vi "mxwScript_API_XMLTemplateName_AddCreateSpace.vi"(8 "error in (no error)":errorcluster, 10 "createSpace?":bool=TRUE, 11 "absolutePath":string) -> (0 "error out":errorcluster, 3 "encoded absolutePath":string)   [LabVIEW 2017]
doc: "Add diagram to drop this template into to the template name."
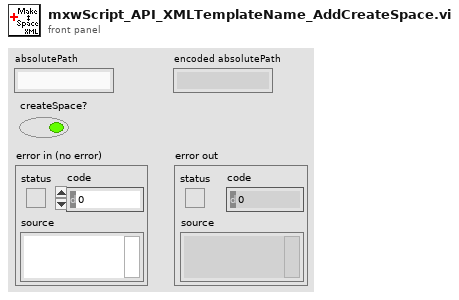
[diagram p1: front panel]
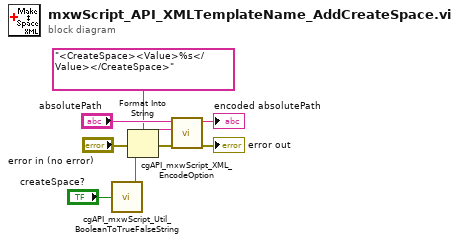
[diagram p0: block diagram]
diagram:
  n1 = call "cgAPI_mxwScript_Util_BooleanToTrueFalseString.vi"("boolean"="createSpace?") -> ("TRUE/FALSE text"=w2:string)  [unwired: 4 out]
  n2 = Format Into String(format string="<CreateSpace><Value>%s</Value></CreateSpace>" ("control name"), error in="error in (no error)", w2) -> (resulting string=w4:string, error out=w6:errorcluster)  [unwired: 1 in]
  n3 = call "cgAPI_mxwScript_XML_EncodeOption.vi"("error in (no error)"=w6, "otherXML"=w4, "normalTextString"="absolutePath") -> ("error out"=→"error out":errorcluster, "encodedString"=→"encoded absolutePath":string)  [unwired: 7 out]
